vi "Check for valid file close.vi"(4 "error in (no error)":errorcluster, 7 "Activity log filepath":path) -> (0 "error out":errorcluster, 2 "Valid Close?":bool)   [LabVIEW 2012]
doc: "Determines if the file has a DIT at the end of the file. If it does not, then add blank DIT string \"<DIT></DIT>\" to file."
panel:
  out "Text at End of File":string
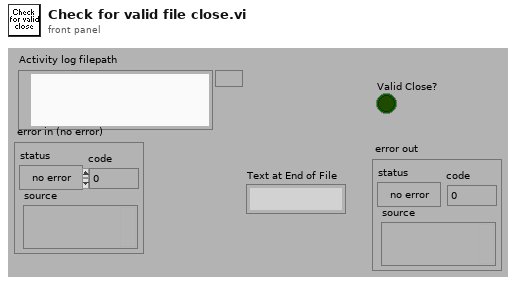
[diagram p1: front panel]
types:
  T1 = enum16{"open", "replace", "create", "open or create", "replace or create", "replace or create with confirmation"}
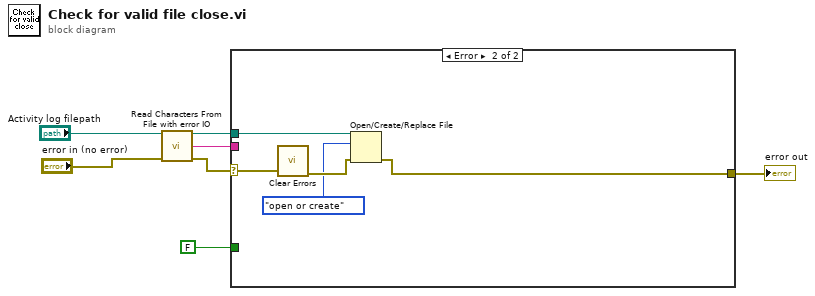
[diagram p0: block diagram]
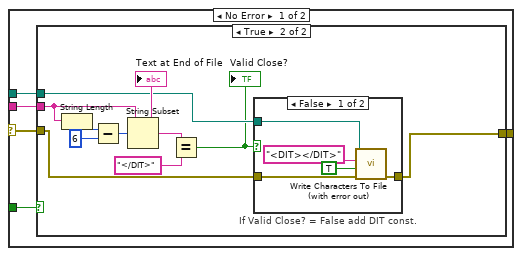
[diagram p2: hidden frame]
diagram:
  n1 = call "Read Characters From File with error IO.vi"("file path (dialog if empty)"="Activity log filepath", "error in (no error)"="error in (no error)") -> ("new file path (NotAPath if cancelled)"=w3:path, "character string"=w4:string, "error out"=w5:errorcluster)  [unwired: 3 in, 8 out]
  n2 = case shown="Error" w5 {
    selector: w5 -> [w10 w34]
    tunnel: w4 -> [w12 _]
    tunnel: w3 -> [w11 w33]
    tunnel: [w9 w31] -> w2
    tunnel: FALSE -> [w8 _]
    frame No Error {
      n3 = case shown="True" w8 {
        tunnel: w12 -> [_ w23]
        tunnel: w11 -> [_ w17]
        tunnel: w10 -> [w13 w16]
        tunnel: [w13 w14] -> w9
        frame False {
        }
        frame True {
          n4 = String Length(string=w23) -> (length=w21:i32)
          n5 = Subtract(x=w21, y=6) -> (x-y=w22:i32)
          n6 = String Subset(string=w23, offset (0)=w22) -> (substring=w19:string)  [unwired: 1 out]
          "Text at End of File" <- w19
          n7 = Equal?(x=w19, y="</DIT>") -> (x = y?=w15:bool)
          "Valid Close?" <- w15
          n8 = case "If Valid Close? = False add DIT const." shown="False" w15 {
            tunnel: w17 -> [w28 _]
            tunnel: w16 -> [w26 w29]
            tunnel: [w24 w29] -> w14
            frame False {
              n9 = call "Write Characters To File (with error out).vi"("error in (no error)"=w26, "append to file? (new file:F)"=TRUE, "character string"="<DIT></DIT>", "file path (dialog if empty)"=w28) -> ("error out"=w24:errorcluster)  [unwired: 3 in, 4 out]
            }
            frame True {
            }
          }
        }
      }
    }
    frame Error {
      n10 = call <vilib>:"Clear Errors.vi"("error in (no error)"=w34) -> ("error out"=w32:errorcluster)  [unwired: 6 out]
      n11 = Open/Create/Replace File(file path (use dialog)=w33, error in=w32, operation (0:open)=T1."open or create") -> (error out=w31:errorcluster)  [unwired: 5 out]
    }
  }
  "error out" <- w2
